vi "Get content in brackets.vi"(6 "TYPE":T1(ring), 10 "start":i32, 11 "String in":string) -> (2 "index out":i32=34, 3 "String out":string)   [LabVIEW 2017, in "API String Arguments Support.lvlib"]
uses:
  API String Arguments Support.lvlib
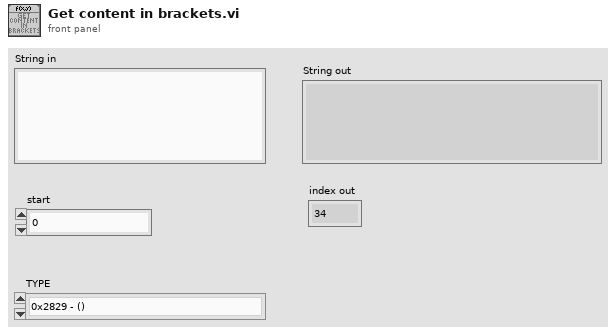
[diagram p1: front panel]
types:
  T1 = enum16{"0x2829 - ()", "0x5B5D - []", "0x7B7D - {}"}
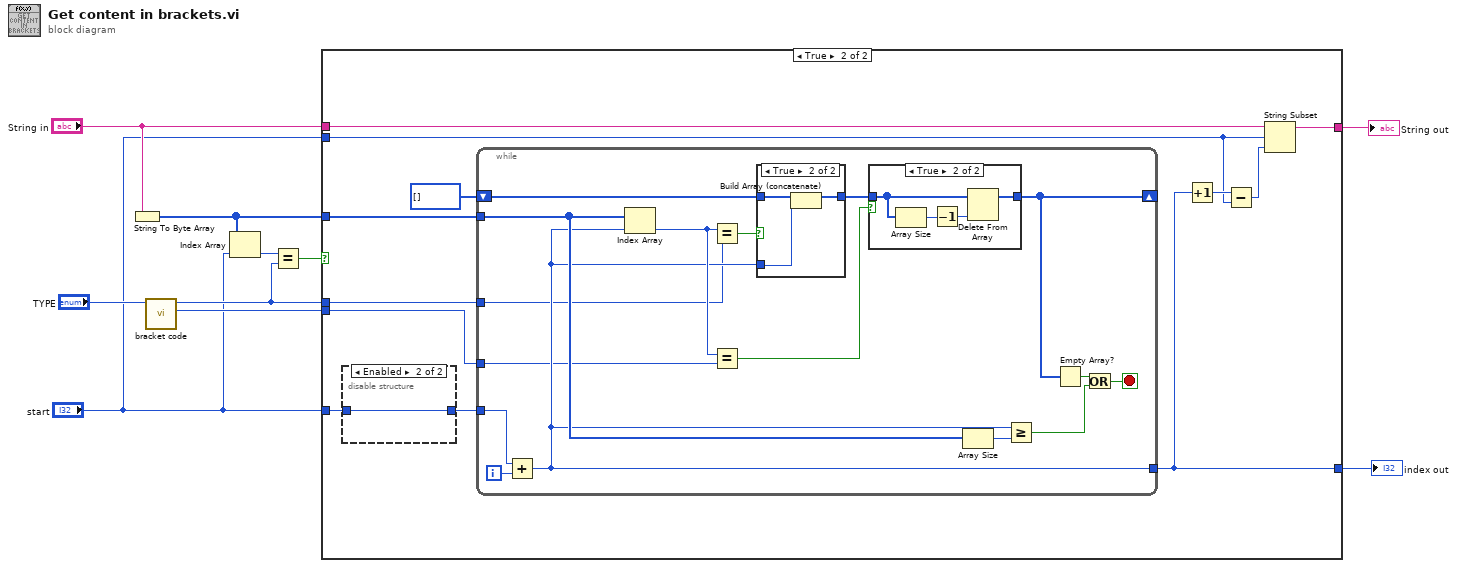
[diagram p0: block diagram]
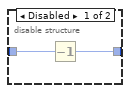
[diagram p3: hidden frame]
diagram:
  n1 = String To Byte Array(string="String in") -> (unsigned byte array=w5:u8[])
  n2 = call "bracket code.vi"("Enum"="TYPE") -> ("Numeric"=w6:u8, "Numeric 2"=w3:u8)  [unwired: 9 in]
  n3 = Index Array(array=w5, index="start") -> (element=w4:u8)
  n4 = Equal?(x=w4, y=w3) -> (x = y?=w2:bool)
  n5 = case shown="True" w2 {
    tunnel: [_ w21] -> w10
    tunnel: [w11 w20] -> w9
    tunnel: "String in" -> [_ w17]
    tunnel: w6 -> [_ w15]
    tunnel: w5 -> [_ w14]
    tunnel: "start" -> [_ w13]
    tunnel: w3 -> [_ w12]
    tunnel: "start" -> [w11 _]
    frame False {
    }
    frame True {
      n6 = disable-structure "Diagram Disable Structure" shown="Enabled" {
        disable-tunnel: w13 -> [w24 w25]
        disable-tunnel: [w23 w25] -> w18
        frame Disabled {
          n7 = Decrement(x=w24) -> (x-1=w23:i32)
        }
        frame Enabled {
        }
      }
      n8 = while {
        tunnel: w14 -> [w30]
        shift-right: [w37] -> _
        shift-left: i32[] [] -> [w32]
        tunnel: [w29] -> w20
        tunnel: w18 -> [w28]
        tunnel: w12 -> [w27]
        tunnel: w15 -> [w26]
        i -> [w31]
        stop <- w36 stop-if-true
        n9 = Add(x=w28, y=w31) -> (x+y=w29:i32)
        n10 = Index Array(array=w30, index=w29) -> (element=w40:u8)
        n11 = Equal?(x=w40, y=w27) -> (x = y?=w41:bool)
        n12 = Equal?(x=w40, y=w26) -> (x = y?=w33:bool)
        n13 = case shown="True" w41 {
          tunnel: w32 -> [w47 w50]
          tunnel: w29 -> [_ w49]
          tunnel: [w47 w48] -> w39
          frame False {
          }
          frame True {
            n14 = Build Array (concatenate)(w50, w49) -> (w48:i32[])
          }
        }
        n15 = case shown="True" w33 {
          tunnel: w39 -> [w42 w45]
          tunnel: [w42 w43] -> w37
          frame False {
          }
          frame True {
            n16 = Array Size(array=w45) -> (size(s)=w46:i32)
            n17 = Decrement(x=w46) -> (x-1=w44:i32)
            n18 = Delete From Array(array=w45, index=w44) -> (array with subset deleted=w43:i32[])  [unwired: 1 in, 1 out]
          }
        }
        n19 = Array Size(array=w30) -> (size(s)=w35:i32)
        n20 = Greater Or Equal?(x=w29, y=w35) -> (x >= y?=w34:bool)
        n21 = Empty Array?(array=w37) -> (empty?=w38:bool)
        n22 = Or(x=w38, y=w34) -> (x .or. y?=w36:bool)
      }
      n23 = Increment(x=w20) -> (x+1=w22:i32)
      n24 = Subtract(x=w22, y=w13) -> (x-y=w19:i32)
      n25 = String Subset(string=w17, offset (0)=w13, length (rest)=w19) -> (substring=w21:string)
    }
  }
  "index out" <- w9
  "String out" <- w10
